vi "String Array Concatenate To String.vi"(7 "insert last delimiter?":bool=TRUE, 10 "Delimiter char":string, 11 "Array String In":string[](array[string])) -> (3 "String":string)   [LabVIEW 2014]
doc: "Concatenates String Array Into one String. If optional delimiter provided, it's inserted between each String Array item. There is option to choose if insert delimiter after last array item, by default yes."
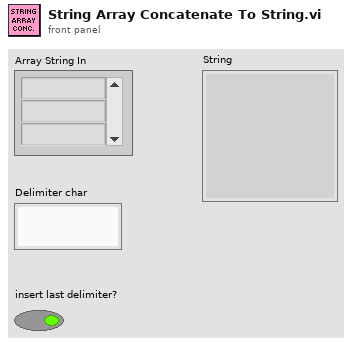
[diagram p1: front panel]
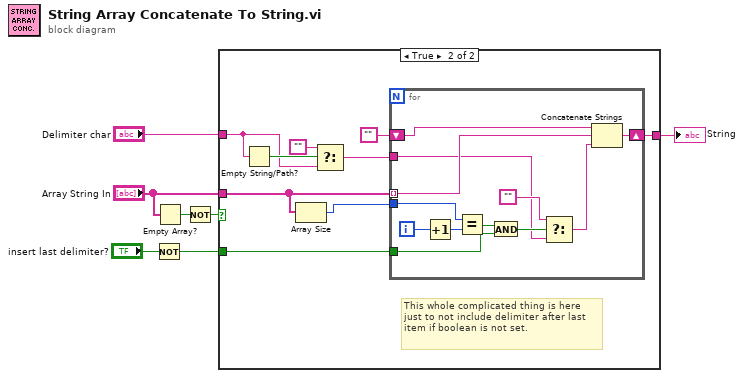
[diagram p0: block diagram]
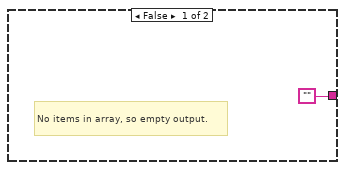
[diagram p2: hidden frame]
diagram:
  n1 = Not(x="insert last delimiter?") -> (.not. x?=w1:bool)
  n2 = Empty Array?(array="Array String In") -> (empty?=w4:bool)
  n3 = Not(x=w4) -> (.not. x?=w2:bool)
  n4 = case shown="True" w2 {
    tunnel: "Delimiter char" -> [_ w15]
    tunnel: ["" w13] -> w6
    tunnel: w1 -> [_ w11]
    tunnel: "Array String In" -> [_ w10]
    frame False {
      # "No items in array, so empty output."
    }
    frame True {
      # "This whole complicated thing is here just to not include delimiter after last item if boolean is not set."
      n5 = Empty String/Path?(string/path=w15) -> (empty?=w17:bool)
      n6 = Array Size(array=w10) -> (size(s)=w9:i32)
      n7 = Select(t="", s=w17, f=w15) -> (s? t:f=w14:string)
      n8 = for {
        tunnel: w10 -> [w27] mode=indexing
        shift-right: [w29] -> w13
        shift-left: "" -> [w28]
        tunnel: w14 -> [w18]
        tunnel: w11 -> [w22]
        tunnel: w9 -> [w24]
        i -> [w26]
        n9 = Increment(x=w26) -> (x+1=w25:i32)
        n10 = Equal?(x=w24, y=w25) -> (x = y?=w23:bool)
        n11 = And(x=w23, y=w22) -> (x .and. y?=w21:bool)
        n12 = Select(t="", s=w21, f=w18) -> (s? t:f=w20:string)
        n13 = Concatenate Strings(w28, w27, w20) -> (w29:string)
      }
    }
  }
  "String" <- w6
